vi "Event to GUI Event.vi"(4 "Event":T2={"Time Stamp"=timestamp(0 s since 1904-01-01), "Event Level"=enum."Info", "Context"="", "Message"="", "Error"={"status"=FALSE, "code"=0, "source"=""}, "Node"=""}, 5 "This Node":string) -> (7 "Event Element":T1)   [LabVIEW 2020, in "VolatusGUI.lvlib" / "Event Viewer Module.lvclass"]
uses:
  Event Viewer Module.lvclass
  Volatus/Event.ctl
  Volatus/Event Level.ctl
  Event Element.ctl
  Event Viewer Module.lvclass/Event Viewer Module.ctl
  Volatus/Volatus.lvlib
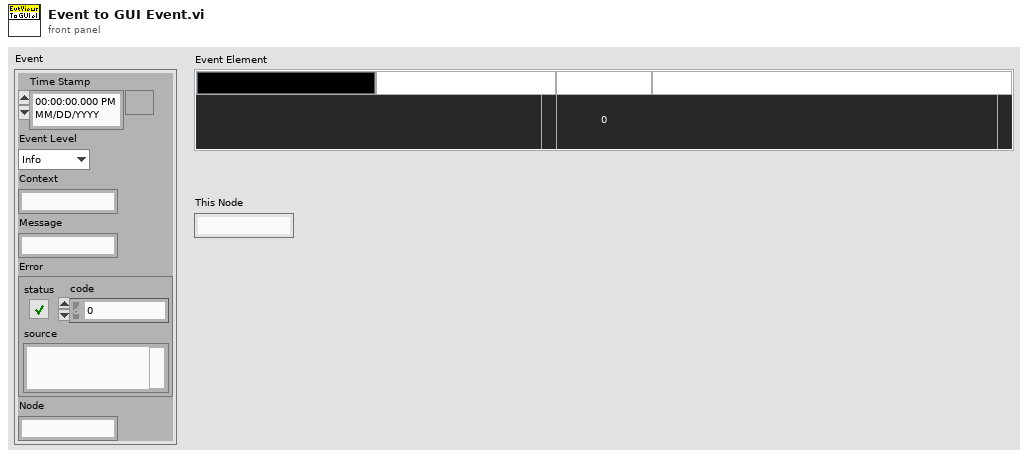
[diagram p1: front panel]
types:
  T1 = typedef "VolatusGUI.lvlib/Event Viewer Module.lvclass/Event Element.ctl" = cluster{"Node":string, "Node Color":u32, "Timestamp":string, "TS Color":u32, "Level":string, "Level Color":u32, "Context":string, "Context Color":u32, "Message":string, "Error Code":i32, "Error Source":string}
  T2 = typedef "Volatus.lvlib/Event.ctl" = cluster{"Time Stamp":timestamp, "Event Level":T3, "Context":string, "Message":string, "Error":errorcluster, "Node":string}
  T3 = typedef "Volatus.lvlib/Event Level.ctl" = enum16{"Debug", "Info", "Warning", "Error"}
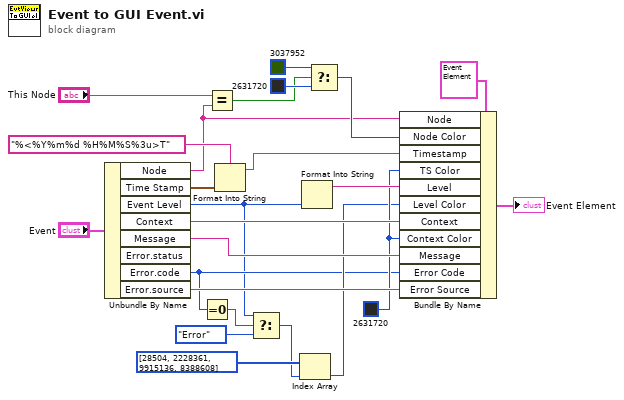
[diagram p0: block diagram]
diagram:
  w15 = u32 2631720 ("System Color")
  n1 = Unbundle By Name("Event") -> ("Node"=w3:string, "Time Stamp"=w22:timestamp, "Event Level"=w9:T3, "Context"=w18:string, "Message"=w17:string, "Error.code"=w11:i32, "Error.source"=w16:string)  [unwired: 1 out]
  n2 = Equal To 0?(x=w11) -> (x = 0?=w10:bool)
  n3 = Equal?(x="This Node", y=w3) -> (x = y?=w1:bool)
  n4 = Format Into String(format string="%<%Y%m%d %H%M%S%3u>T", w22) -> (resulting string=w20:string)  [unwired: 2 in, 1 out]
  n5 = Select(t=w9, s=w10, f=Event_Level."Error") -> (s? t:f=w7:T3)
  n6 = Index Array(array=u32[] [28504, 2228361, 9915136, 8388608], index=w7) -> (element=w12:u32)
  n7 = Format Into String(w9) -> (resulting string=w19:string)  [unwired: 3 in, 1 out]
  n8 = Select(t=u32 3037952, s=w1, f=u32 2631720) -> (s? t:f=w4:u32)
  n9 = Bundle By Name(cluster=T1 {"Node"="", "Node Color"=2631720, "Timestamp"="YYYYMMDD 000000.000", "TS Color"=2631720, "Level"="", "Level Color"=2631720, "Context"="", "Context Color"=2631720, "Message"="", "Error Code"=-2147483648, "Error Source"=""} ("Event Element"), "Node"=w3, "Node Color"=w4, "Timestamp"=w20, "TS Color"=w15, "Level"=w19, "Level Color"=w12, "Context"=w18, "Context Color"=w15, "Message"=w17, "Error Code"=w11, "Error Source"=w16) -> (→"Event Element":T1)
